vi "get calibration settings.vi"(8 "error in (no error)":errorcluster, 10 "calibration_settings":T1, 11 "id":i32) -> (0 "error out":errorcluster, 2 "calibration_settings out":T1, 3 "function return":i32)   [LabVIEW 2012, in "libximc.lvlib"]
doc: "result_t XIMC_API get_calibration_settings (device_t id, calibration_settings_t* calibration_settings);"
uses:
  libximc.lvlib
  libximc.dll
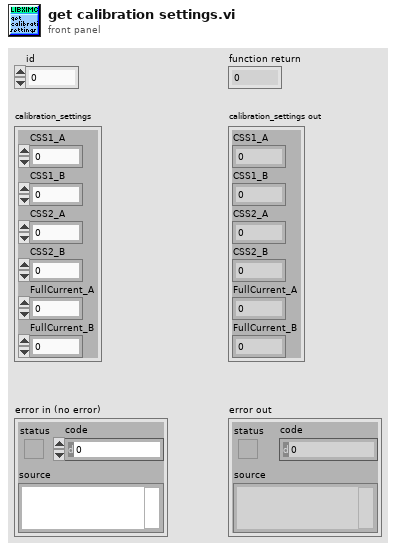
[diagram p1: front panel]
types:
  T1 = cluster{"CSS1_A":sgl, "CSS1_B":sgl, "CSS2_A":sgl, "CSS2_B":sgl, "FullCurrent_A":sgl, "FullCurrent_B":sgl}
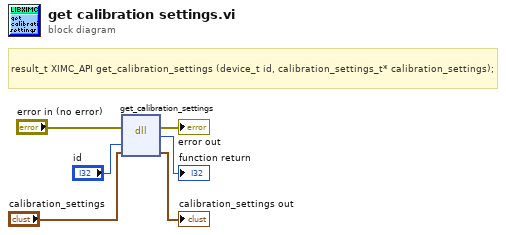
[diagram p0: block diagram]
diagram:
  # "result_t XIMC_API get_calibration_settings (device_t id, calibration_settings_t* calibration_settings);"
  n1 = dll-call lib="E:/labview-2.12.1-Labview_12.0/ximcLVx32/libximc.*" fn="get_calibration_settings"(error in="error in (no error)", "id"="id", "calibration_settings"="calibration_settings") -> (error out=→"error out":errorcluster, →"function return":i32, "calibration_settings"=→"calibration_settings out":T1)  [unwired: 3 in, 1 out]
